vi "Create Remote File.vi"(8 "Error In":errorcluster, 10 "Remote Path In":string, 11 "SFTP In":refnum<class "SFTP.lvclass">) -> (0 "Error Out":errorcluster, 2 "Remote Path Out":string, 3 "SFTP Out":refnum<class "SFTP.lvclass">)   [LabVIEW 2018, in "Tests.lvlib" / "SFTP File.lvlib"]
uses:
  SFTP File.lvlib
  src/Toolkit/SFTP/SFTP.lvclass
  src/Toolkit/SFTP File/Type Definitions/Flags.ctl
  src/Toolkit/Type Definitions/Permissions.ctl
  src/Toolkit/Type Definitions/Modes.ctl
  src/Toolkit/SFTP File/SFTP File.lvclass
  src/Toolkit/Toolkit.lvlib
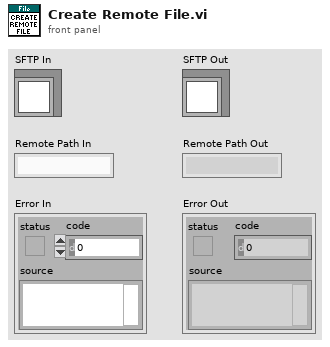
[diagram p1: front panel]
types:
  T1 = enum16{"open", "replace", "create", "open or create", "replace or create", "replace or create with confirmation"}
  T2 = typedef "Toolkit.lvlib/Permissions.ctl" = cluster{"Owner":T3, "Group":T3, "Others":T3}
  T3 = typedef "Toolkit.lvlib/Modes.ctl" = cluster{"Read":bool, "Write":bool, "Execute":bool}
  T4 = typedef "Toolkit.lvlib/SFTP File.lvclass/Flags.ctl" = cluster{"Read":bool, "Write":bool, "Append":bool, "Create":bool, "Truncate":bool, "Exclude":bool}
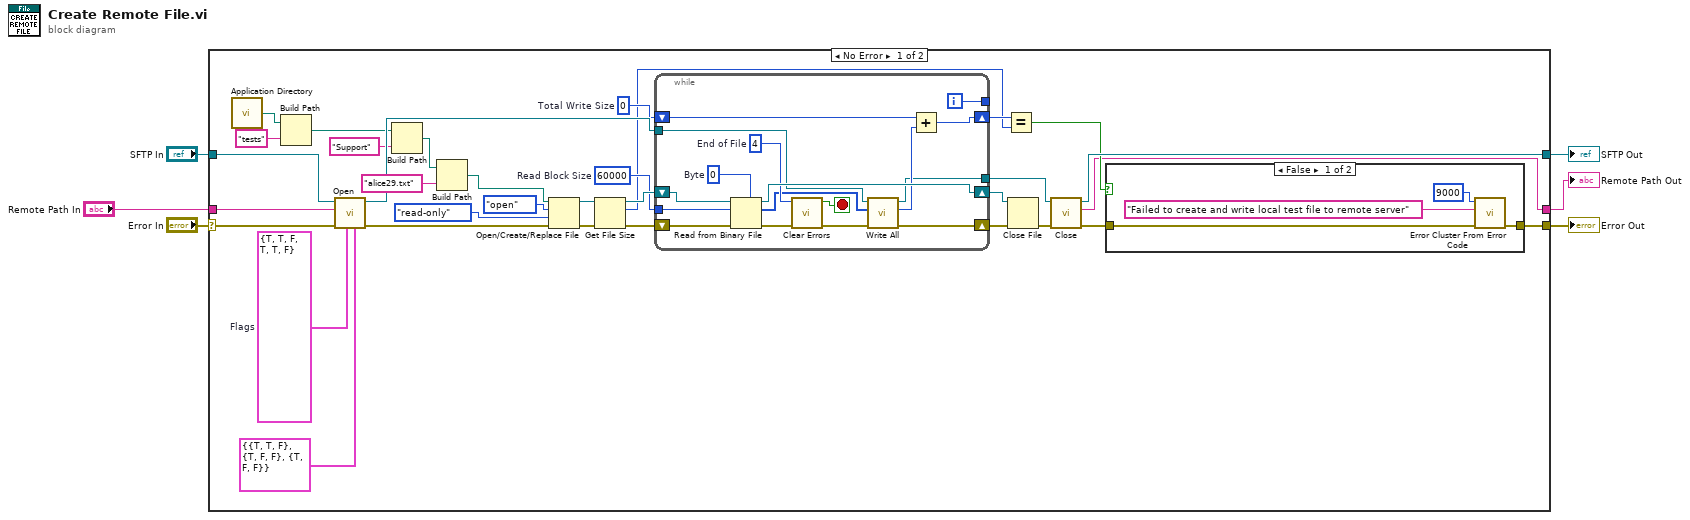
[diagram p0: block diagram]
diagram:
  n1 = case shown="No Error" "Error In" {
    selector: "Error In" -> [w8 w63]
    tunnel: [w16 w64] -> w6
    tunnel: "SFTP In" -> [w15 w64]
    tunnel: "Remote Path In" -> [w14 w62]
    tunnel: [w9 w63] -> w3
    tunnel: [w7 w62] -> w1
    frame No Error {
      w19 = i64 60000  # Read Block Size
      w23 = i64 0  # Total Write Size
      w38 = T4 {"Read"=TRUE, "Write"=TRUE, "Append"=FALSE, "Create"=TRUE, "Truncate"=TRUE, "Exclude"=FALSE}  # Flags
      n2 = call <vilib>:"Application Directory.vi"() -> ("Application Directory"=w33:path)
      n3 = Build Path(base path=w33, name or relative path="tests") -> (appended path=w31:path)
      n4 = call "Open.vi"("Permissions"=T2 {"Owner"={"Read"=TRUE, "Write"=TRUE, "Execute"=FALSE}, "Group"={"Read"=TRUE, "Write"=FALSE, "Execute"=FALSE}, "Others"={"Read"=TRUE, "Write"=FALSE, "Execute"=FALSE}}, "Flags"=w38, "Error In"=w8, "Remote Path"=w14, "SFTP"=w15) -> ("Error Out"=w24:errorcluster, "SFTP File"=w39:refnum<class "SFTP File.lvclass">)  [unwired: 5 in]
      n5 = Build Path(base path=w31, name or relative path="Support") -> (appended path=w29:path)
      n6 = Build Path(base path=w29, name or relative path="alice29.txt") -> (appended path=w28:path)
      n7 = Open/Create/Replace File(file path (use dialog)=w28, error in=w24, operation (0:open)=T1."open", access (0:read/write)=enum16{"read/write", "read-only", "write-only"}."read-only") -> (refnum out=w34:refnum<file>, error out=w21:errorcluster)  [unwired: 2 in, 1 out]
      n8 = Get File Size(file=w34, error in=w21) -> (refnum out=w22:refnum<file>, size (in bytes)=w12:i64, 0:w20:errorcluster)
      n9 = while {
        tunnel: w39 -> [w46]
        tunnel: w19 -> [w52]
        shift-right: [w59] -> w27
        shift-left: w22 -> [w61]
        shift-right: [w49] -> w26
        shift-left: w20 -> [w60]
        tunnel: [w47] -> w18
        shift-right: [w53] -> w13
        shift-left: w23 -> [w56]
        tunnel: [w54] -> _
        i -> [w54]
        stop <- w51 stop-if-true
        w55 = u8 0  # Byte
        w57 = 4  # End of File
        n10 = Read from Binary File(5:w55, 8:w60, 10:w52, 11:w61) -> (0:w58:errorcluster, 2:w45:u8[], 3:w59:refnum<file>)  [unwired: 2 in, 1 out]
        n11 = call <vilib>:"Clear Errors.vi"("error in (no error)"=w58, "specific error code to clear (0: all)"=w57) -> ("error out"=w50:errorcluster, "specific error cleared?"=w51:bool)  [unwired: 4 in]
        n12 = call "Write All.vi"("Error In"=w50, "Bytes"=w45, "SFTP File In"=w46) -> ("Error Out"=w49:errorcluster, "Block Write Count"=w48:i64, "SFTP File Out"=w47:refnum<class "SFTP File.lvclass">)  [unwired: 6 in]
        n13 = Add(x=w56, y=w48) -> (x+y=w53:i64)
      }
      n14 = Equal?(x=w13, y=w12) -> (x = y?=w11:bool)
      n15 = Close File(refnum=w27, error in=w26) -> (error out=w17:errorcluster)  [unwired: 1 out]
      n16 = call "Close.vi"("Error In"=w17, "SFTP File"=w18) -> ("Error Out"=w10:errorcluster, "Remote Path"=w7:string, "SFTP"=w16:refnum<class "SFTP.lvclass">)  [unwired: 7 in]
      n17 = case shown="False" w11 {
        tunnel: w10 -> [w43 w44]
        tunnel: [w42 w44] -> w9
        frame False {
          n18 = call <vilib>:"Error Cluster From Error Code.vi"("error in (no error)"=w43, "error message (\"\")"="Failed to create and write local test file to remote server" ("error message (\"\")"), "error code (0)"=9000) -> ("error out"=w42:errorcluster)  [unwired: 6 in]
        }
        frame True {
        }
      }
    }
    frame Error {
    }
  }
  "Error Out" <- w3
  "SFTP Out" <- w6
  "Remote Path Out" <- w1
